vi "預防保養設定次數To PLC_2.vi"(9 "Set Value Or Only Read":bool, 10 "Out starting address":u16=300, 11 "Input Registers":u16[](array[numeric])=[0, 0, 0, 0, 0, 0, 0, 0]) -> (0 "error out":errorcluster, 2 "預防保養實際數":i32[](array[numeric]), 3 "預防保養設定次數顯示":i32[](array[numeric]))   [LabVIEW 2019]
panel:
  out "Array":string[](array[string])
  out "String":string
  in  "subarray 4":string[](array[string])=["S1-檢平確認氣缸 (設定值)", "$S1_PreventionChk 1", "S1 電路板檢平On次數(設定值)", "$S1_PreventionChk 2", "S1 電池檢平On次數(設定值)", "$S1_PreventionChk 3", "S1 盒蓋檢平On次數(設定值)", "$S1_PreventionChk 4", "S2電流量測 探針使用次數(設定值)", "$S2_PreventionChk 1", "S2-電流量測氣缸 (設定值)", "$S2_PreventionChk 2", "S3程式燒入 探針使用次數(設定值)", "$S3_PreventionChk 1", "S3-程式燒入氣缸 (設定值)", "$S3_PreventionChk 2", "S4電壓量測探針使用次數(設定值)", "$S4_PreventionChk 1", "S4電源3V探針使用次數(設定值)", "$S4_PreventionChk 2", "S4 隔離箱上蓋氣缸 (設定值)", "$S4_PreventionChk 3", "S4 隔離箱下蓋氣缸 (設定值)", "$S4_PreventionChk 4", "S4 電池電壓量測固定氣缸 (設定值)", "$S4_PreventionChk 5", "S4 電池電壓量測氣缸 (設定值)", "$S4_PreventionChk 6", "S4 電路板檢測氣缸(設定值)", "$S4_PreventionChk 7", "S5 電路板取料升降氣缸 (設定值)", "$S5_PreventionChk 1", "S5 電路板取料橫移氣缸 (設定值)", "$S5_PreventionChk 2", "S5 真空 吸取(設定值)", "$S5_PreventionChk 3", "S5 真空 解除(設定值)", "$S5_PreventionChk 4", "S7 焊接料件固定氣缸 (設定值)", "$S7_PreventionChk 1", "S7 焊接機清錫馬達 (設定值)", "$S7_PreventionChk 2", "S10 料件翻轉區升降氣缸 (設定值)", "$S10_PreventionChk 1", "S10 料件翻轉區伸出氣缸 (設定值)", "$S10_PreventionChk 2", "S10 料件翻轉區旋轉氣缸 (設定值)", "$S10_PreventionChk 3", "S10 料件翻轉區夾取氣缸 (設定值)", "$S10_PreventionChk 4", "S10 料件橫移氣缸 (設定值)", "$S10_PreventionChk 5", "S10 料件吸取升降氣缸 (設定值)", "$S10_PreventionChk 6", "S10 料件放料升降氣缸 (設定值)", "$S10_PreventionChk 7", "S10 真空 吸取(設定值)", "$S10_PreventionChk 8", "S10 真空 解除(設定值)", "$S10_PreventionChk 9", "S11 雷射測高檢知氣缸 (設定值)", "$S11_PreventionChk 1", "S12 熱熔升降氣缸 (設定值)", "$S12_PreventionChk 1", "S12 預熱升降氣缸 (設定值)", "$S12_PreventionChk 2", "S12 離子槍風速調控 (設定值)", "$S12_PreventionChk 3", "S13 真空 吸取 (設定值)", "$S13_PreventionChk 1", "S13 真空 解除(設定值)", "$S13_PreventionChk 2", "S13 NG蓋取料夾爪 (設定值)", "$S13_PreventionChk 3", "S13 NG蓋取料升降 (設定值)", "$S13_PreventionChk 4", "S13 NG電池取料升降 (設定值)", "$S13_PreventionChk 5", "S13 NG電路板取料升降 (設定值)", "$S13_PreventionChk 6", "S13 NG橫移氣缸 (設定值)", "$S13_PreventionChk 7", "S13 NG橫移氣缸(設定值)", "$S13_PreventionChk 8", "S7 焊接啟動次數(設定值)", "$S7_PreventionChk 1", "S12 熱熔次數(設定值)", "$S12_PreventionChk 4", "S11 雷射檢測次數(設定值)", "$S11_PreventionChk 1"]
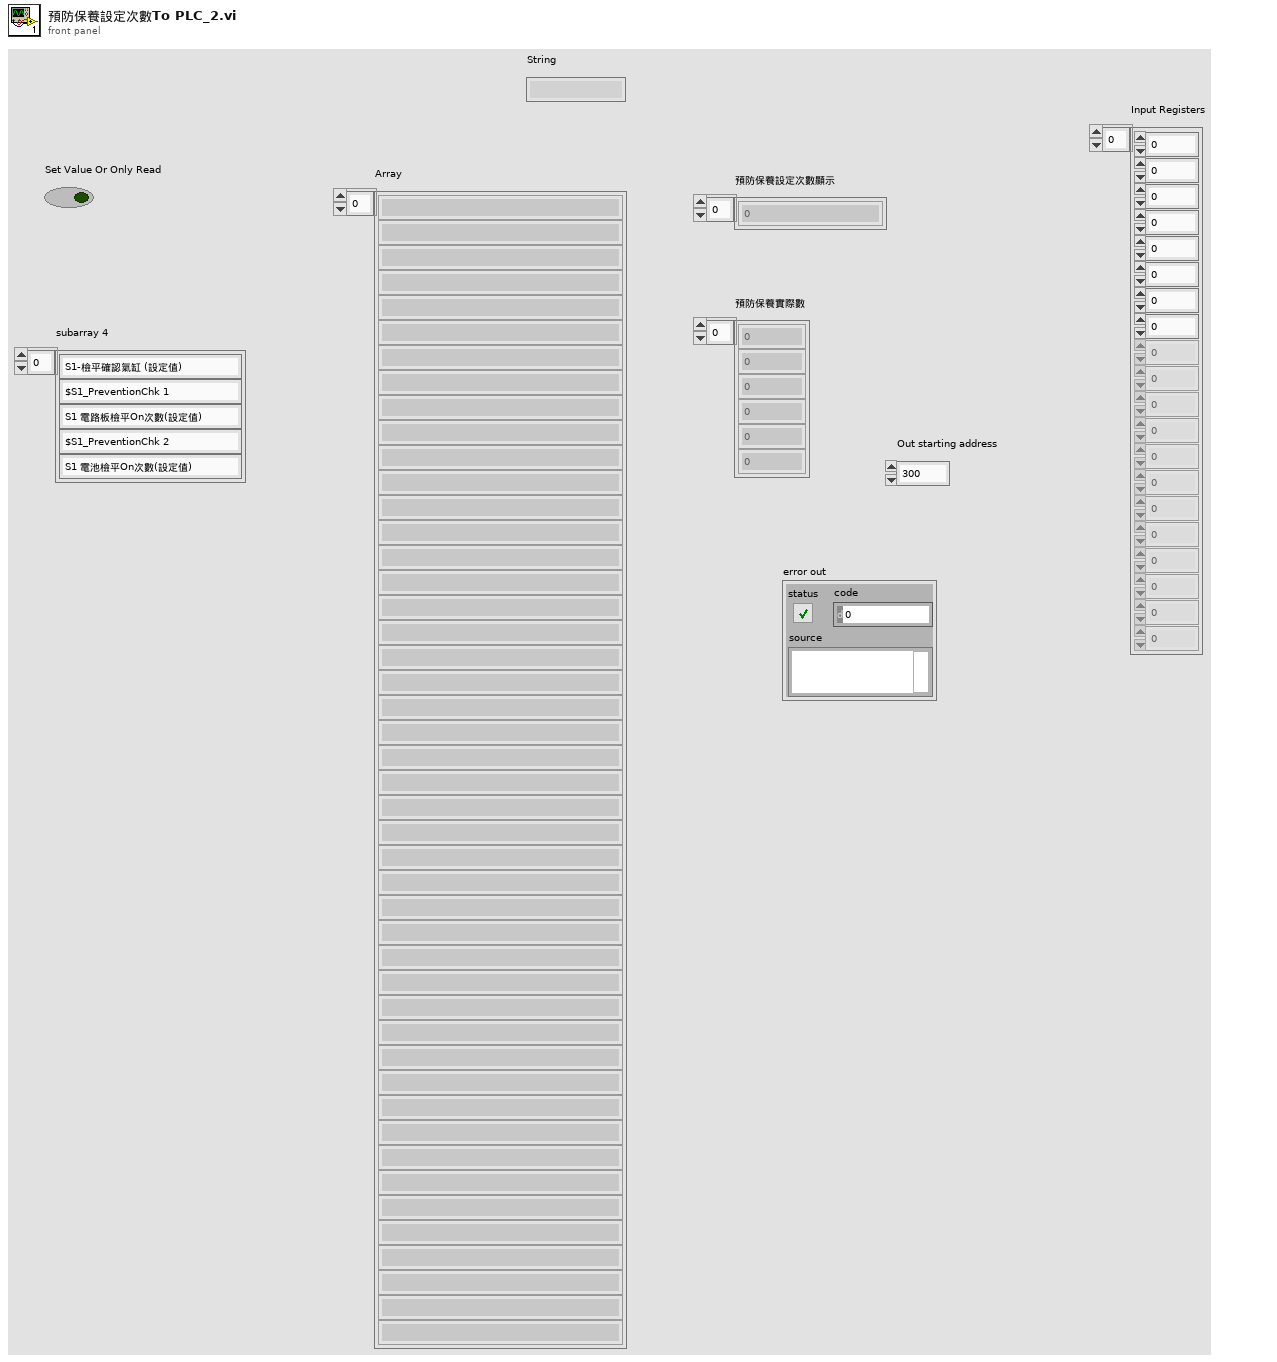
[diagram p1: front panel]
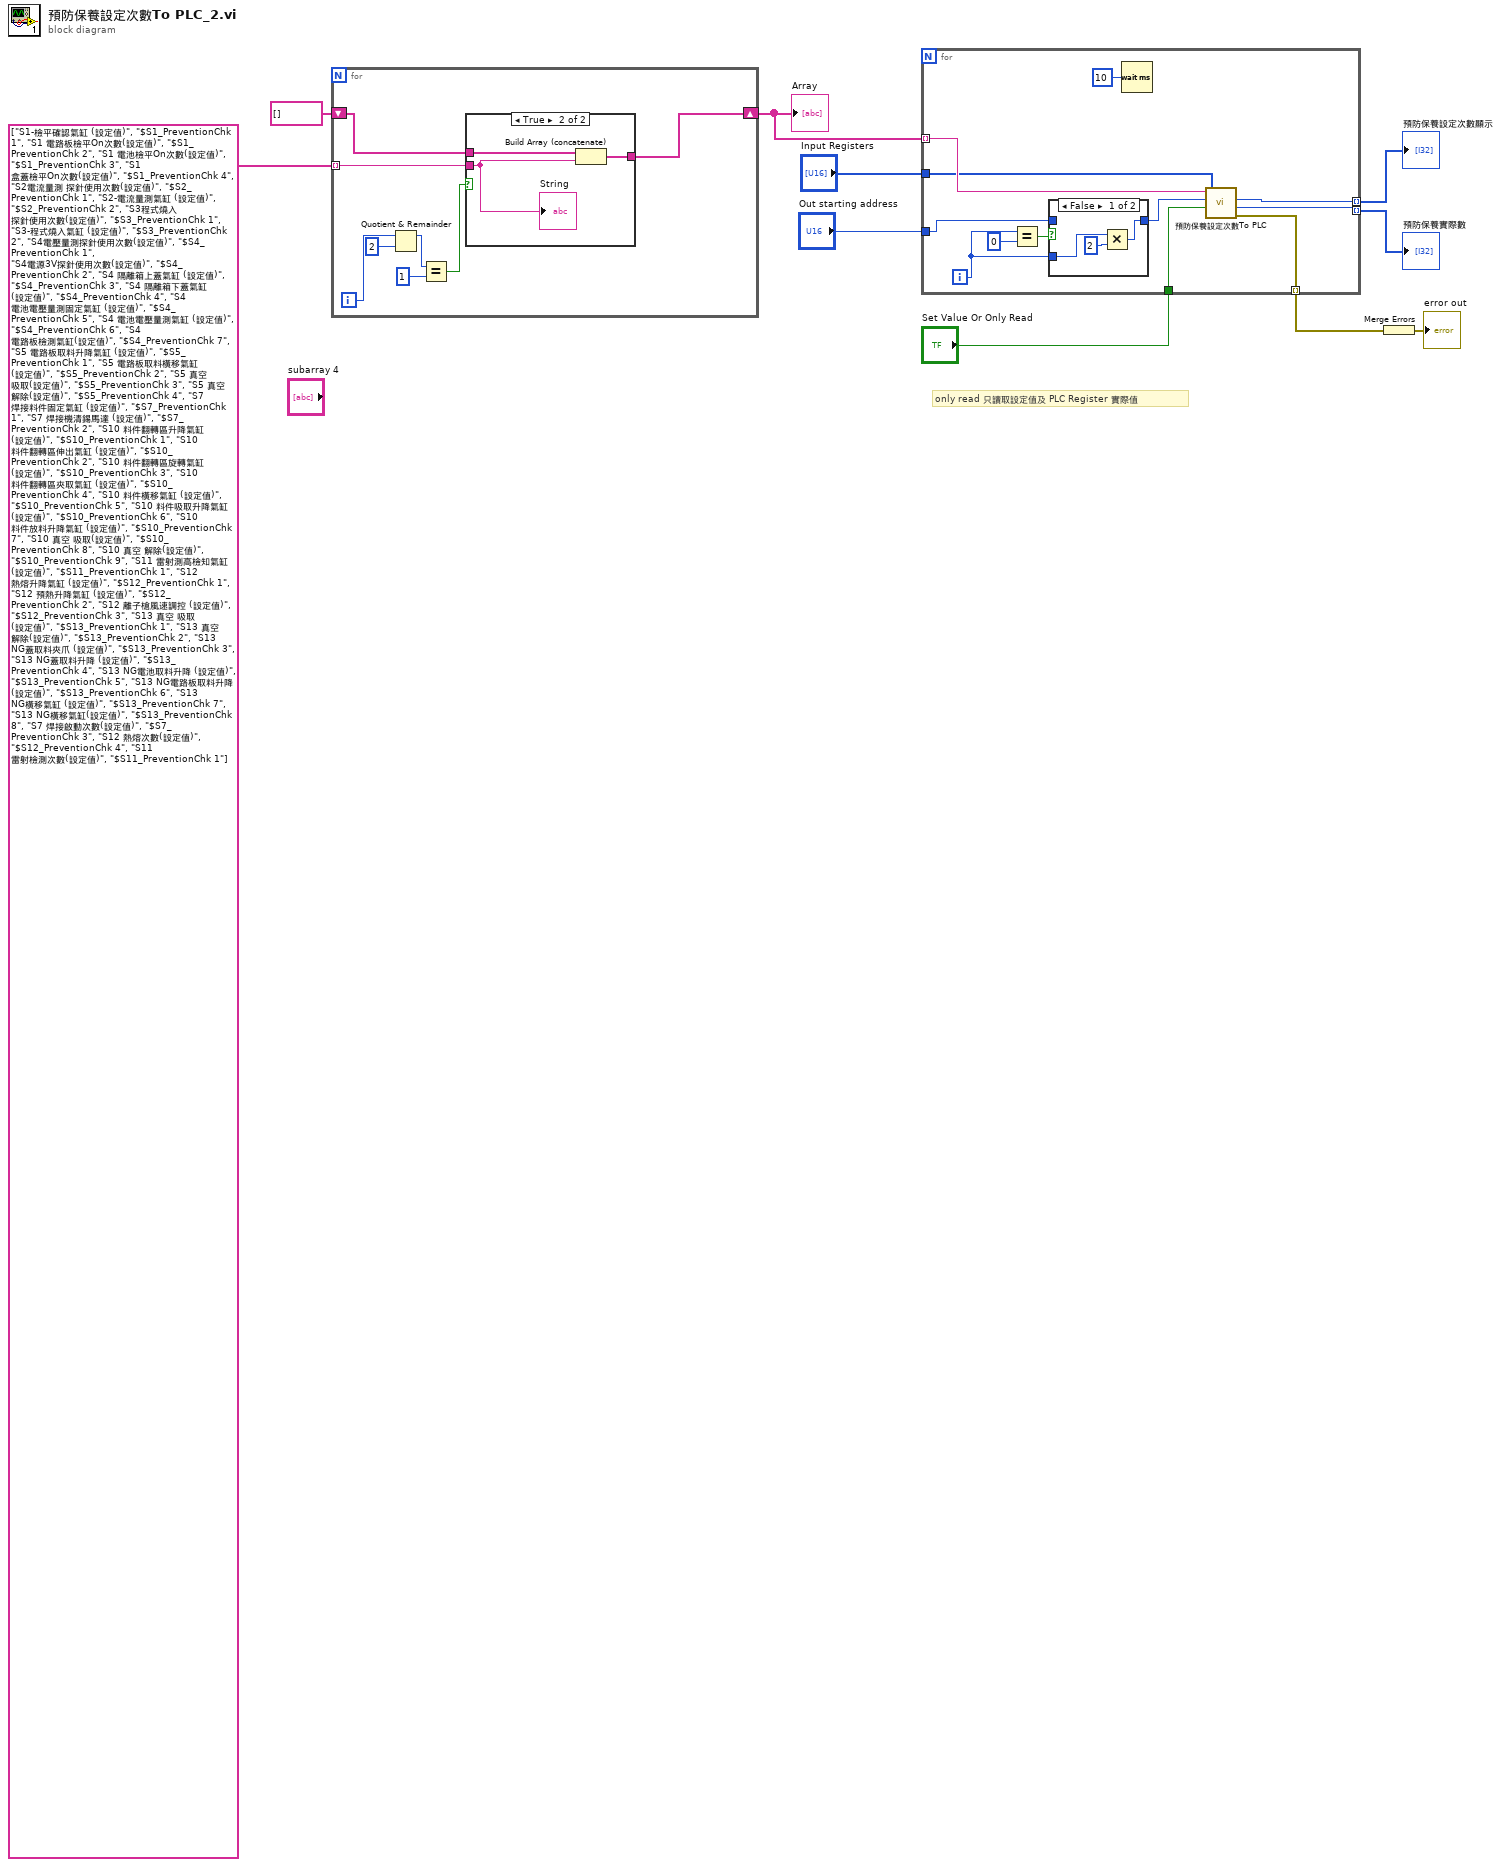
[diagram p0: block diagram]
diagram:
  # "only read 只讀取設定值及 PLC Register 實際值"
  n1 = for {
    tunnel: string[] ["S1-檢平確認氣缸 (設定值)", "$S1_PreventionChk 1", "S1 電路板檢平On次數(設定值)", "$S1_PreventionChk 2", "S1 電池檢平On次數(設定值)", "$S1_PreventionChk 3", "S1 盒蓋檢平On次數(設定值)", "$S1_PreventionChk 4", "S2電流量測 探針使用次數(設定值)", "$S2_PreventionChk 1", "S2-電流量測氣缸 (設定值)", "$S2_PreventionChk 2", "S3程式燒入 探針使用次數(設定值)", "$S3_PreventionChk 1", "S3-程式燒入氣缸 (設定值)", "$S3_PreventionChk 2", "S4電壓量測探針使用次數(設定值)", "$S4_PreventionChk 1", "S4電源3V探針使用次數(設定值)", "$S4_PreventionChk 2", "S4 隔離箱上蓋氣缸 (設定值)", "$S4_PreventionChk 3", "S4 隔離箱下蓋氣缸 (設定值)", "$S4_PreventionChk 4", "S4 電池電壓量測固定氣缸 (設定值)", "$S4_PreventionChk 5", "S4 電池電壓量測氣缸 (設定值)", "$S4_PreventionChk 6", "S4 電路板檢測氣缸(設定值)", "$S4_PreventionChk 7", "S5 電路板取料升降氣缸 (設定值)", "$S5_PreventionChk 1", "S5 電路板取料橫移氣缸 (設定值)", "$S5_PreventionChk 2", "S5 真空 吸取(設定值)", "$S5_PreventionChk 3", "S5 真空 解除(設定值)", "$S5_PreventionChk 4", "S7 焊接料件固定氣缸 (設定值)", "$S7_PreventionChk 1", "S7 焊接機清錫馬達 (設定值)", "$S7_PreventionChk 2", "S10 料件翻轉區升降氣缸 (設定值)", "$S10_PreventionChk 1", "S10 料件翻轉區伸出氣缸 (設定值)", "$S10_PreventionChk 2", "S10 料件翻轉區旋轉氣缸 (設定值)", "$S10_PreventionChk 3", "S10 料件翻轉區夾取氣缸 (設定值)", "$S10_PreventionChk 4", "S10 料件橫移氣缸 (設定值)", "$S10_PreventionChk 5", "S10 料件吸取升降氣缸 (設定值)", "$S10_PreventionChk 6", "S10 料件放料升降氣缸 (設定值)", "$S10_PreventionChk 7", "S10 真空 吸取(設定值)", "$S10_PreventionChk 8", "S10 真空 解除(設定值)", "$S10_PreventionChk 9", "S11 雷射測高檢知氣缸 (設定值)", "$S11_PreventionChk 1", "S12 熱熔升降氣缸 (設定值)", "$S12_PreventionChk 1", "S12 預熱升降氣缸 (設定值)", "$S12_PreventionChk 2", "S12 離子槍風速調控 (設定值)", "$S12_PreventionChk 3", "S13 真空 吸取 (設定值)", "$S13_PreventionChk 1", "S13 真空 解除(設定值)", "$S13_PreventionChk 2", "S13 NG蓋取料夾爪 (設定值)", "$S13_PreventionChk 3", "S13 NG蓋取料升降 (設定值)", "$S13_PreventionChk 4", "S13 NG電池取料升降 (設定值)", "$S13_PreventionChk 5", "S13 NG電路板取料升降 (設定值)", "$S13_PreventionChk 6", "S13 NG橫移氣缸 (設定值)", "$S13_PreventionChk 7", "S13 NG橫移氣缸(設定值)", "$S13_PreventionChk 8", "S7 焊接啟動次數(設定值)", "$S7_PreventionChk 3", "S12 熱熔次數(設定值)", "$S12_PreventionChk 4", "S11 雷射檢測次數(設定值)", "$S11_PreventionChk 1"] ("subarray 6") -> [w13] mode=indexing
    shift-right: [w12] -> w8
    shift-left: string[] [] -> [w11]
    i -> [w18]
    n2 = Quotient & Remainder(x=w18, y=2) -> (x-y*floor(x/y)=w16:i32)  [unwired: 1 out]
    n3 = Equal?(x=w16, y=1) -> (x = y?=w14:bool)
    n4 = case shown="True" w14 {
      tunnel: w13 -> [_ w22]
      tunnel: [w19 w21] -> w12
      tunnel: w11 -> [w19 w20]
      frame False {
      }
      frame True {
        n5 = Build Array (concatenate)(w20, w22) -> (w21:string[])
        "String" <- w22
      }
    }
  }
  "Array" <- w8
  n6 = for {
    tunnel: w8 -> [w32] mode=indexing
    tunnel: [w33] -> w7 mode=indexing
    tunnel: "Out starting address" -> [w26]
    tunnel: "Set Value Or Only Read" -> [w31]
    tunnel: [w30] -> w4 mode=indexing
    tunnel: "Input Registers" -> [w29]
    tunnel: [w23] -> w2 mode=indexing
    i -> [w24]
    n7 = Equal?(x=w24, y=0) -> (x = y?=w28:bool)
    n8 = case shown="False" w28 {
      tunnel: w26 -> [_ w38]
      tunnel: [w37 w38] -> w25
      tunnel: w24 -> [w36 _]
      frame False {
        n9 = Multiply(x=w36, y=2) -> (x*y=w37:i32)
      }
      frame True {
      }
    }
    n10 = Wait (ms)(milliseconds to wait=u32 10) -> ()  [unwired: 1 out]
    n11 = call "預防保養設定次數To PLC.vi"("Input Registers"=w29, "Set Value Or Only Read"=w31, "Out starting address"=w25, "Set Item"=w32) -> ("error out"=w23:errorcluster, "Receive PLC Data"=w30:i32, "data"=w33:i32)  [unwired: 5 in]
  }
  "預防保養設定次數顯示" <- w7
  "預防保養實際數" <- w4
  n12 = Merge Errors(w2) -> (→"error out":errorcluster)
